vi "Create File Name (SubVI).vi"(1 "Extension":string=".raw", 2 "File Name Prefix":string="Rawdata ", 3 "File Path":path) -> (4 "File Name":path)   [LabVIEW 2015]
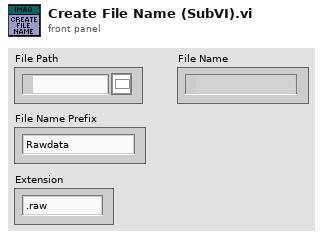
[diagram p1: front panel]
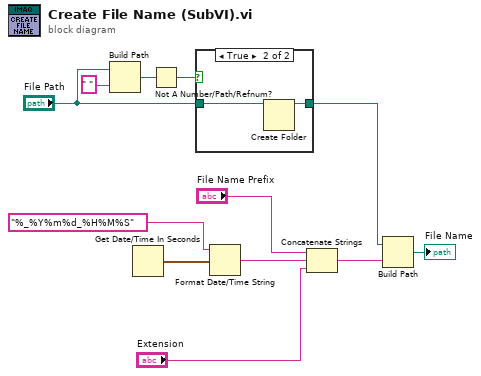
[diagram p0: block diagram]
diagram:
  n1 = Build Path(base path="File Path", name or relative path=" ") -> (appended path=w7:path)
  n2 = Get Date/Time In Seconds() -> (seconds since 1Jan1904=w4:timestamp)
  n3 = Not A Number/Path/Refnum?(number/path/refnum=w7) -> (NaN/Path/Refnum?=w10:bool)
  n4 = case shown="True" w10 {
    tunnel: "File Path" -> [w13 w15]
    tunnel: [w13 w14] -> w11
    frame False {
    }
    frame True {
      n5 = Create Folder(path (use dialog)=w15) -> (created path=w14:path)  [unwired: 2 in, 2 out]
    }
  }
  n6 = Format Date/Time String(time format string (%c)="%_%Y%m%d_%H%M%S", seconds (now)=w4) -> (date/time string=w1:string)  [unwired: 1 in]
  n7 = Concatenate Strings("File Name Prefix", w1, "Extension") -> (w9:string)
  n8 = Build Path(base path=w11, name or relative path=w9) -> (appended path=→"File Name":path)
